vi "subAcquisition_zStack.vi"(6 "Ti-E cluster":T2, 7 "Z-stack cluster":T1={"Timelapse Acquired"=1, "File path"=path "C:/Users/ZouOptics/Desktop/TEST", "Z-Stack"={"Z end"=0.0, "Step Num"=1, "Step Size"=2.0, "Z0"=3471.0, "z-stack?"=FALSE}, "Frames to avg."=20, "Image Info Ref"=refnum, "Camera Ctrl"={"Chosen Camera"=0, "ROI selection"=0, "Live"=FALSE, "ROI define"=FALSE, "Snap"=FALSE, "ROI update"=FALSE, "ROI previous "=FALSE, "ROI"={"Bin"=2, "ROI"={"x offset"=256, "y offset"=256, "x width"=512, "y width"=512}}, "Exposure (ms)"=100.0, "Symmetrical"=FALSE, "Autoscale"=TRUE, "Scale"={"Scale.Min"=0, "Scale.Max"=6038}}} {"Camera Ctrl"."Scale"."Scale.Max" min=1 max=5000 step=1; "Camera Ctrl"."Scale"."Scale.Min" min=1 max=5000 step=1; "Camera Ctrl"."Exposure (ms)" min=1.0 max=5000.0 step=1.0; "Camera Ctrl"."ROI"."ROI"."x offset" min=1 max=512 step=1; "Camera Ctrl"."ROI"."ROI"."y offset" min=1 max=512 step=1; "Camera Ctrl"."ROI"."ROI"."x width" min=1 max=512 step=1; "Camera Ctrl"."ROI"."ROI"."y width" min=1 max=512 step=1; "Camera Ctrl"."ROI"."Bin" items=["1x1"=1, "2x2"=2, "4x4"=4]; "Camera Ctrl"."ROI selection" items=["Full ROI", "Central quad", "Confocal"]; "Camera Ctrl"."Chosen Camera" items=["Left", "Right"]}, 8 "error in":errorcluster, 10 "Z Stack Aquired Refnum":refnum<vi>, 11 "Handle in":u32) -> (0 "error out":errorcluster)   [LabVIEW 2015]
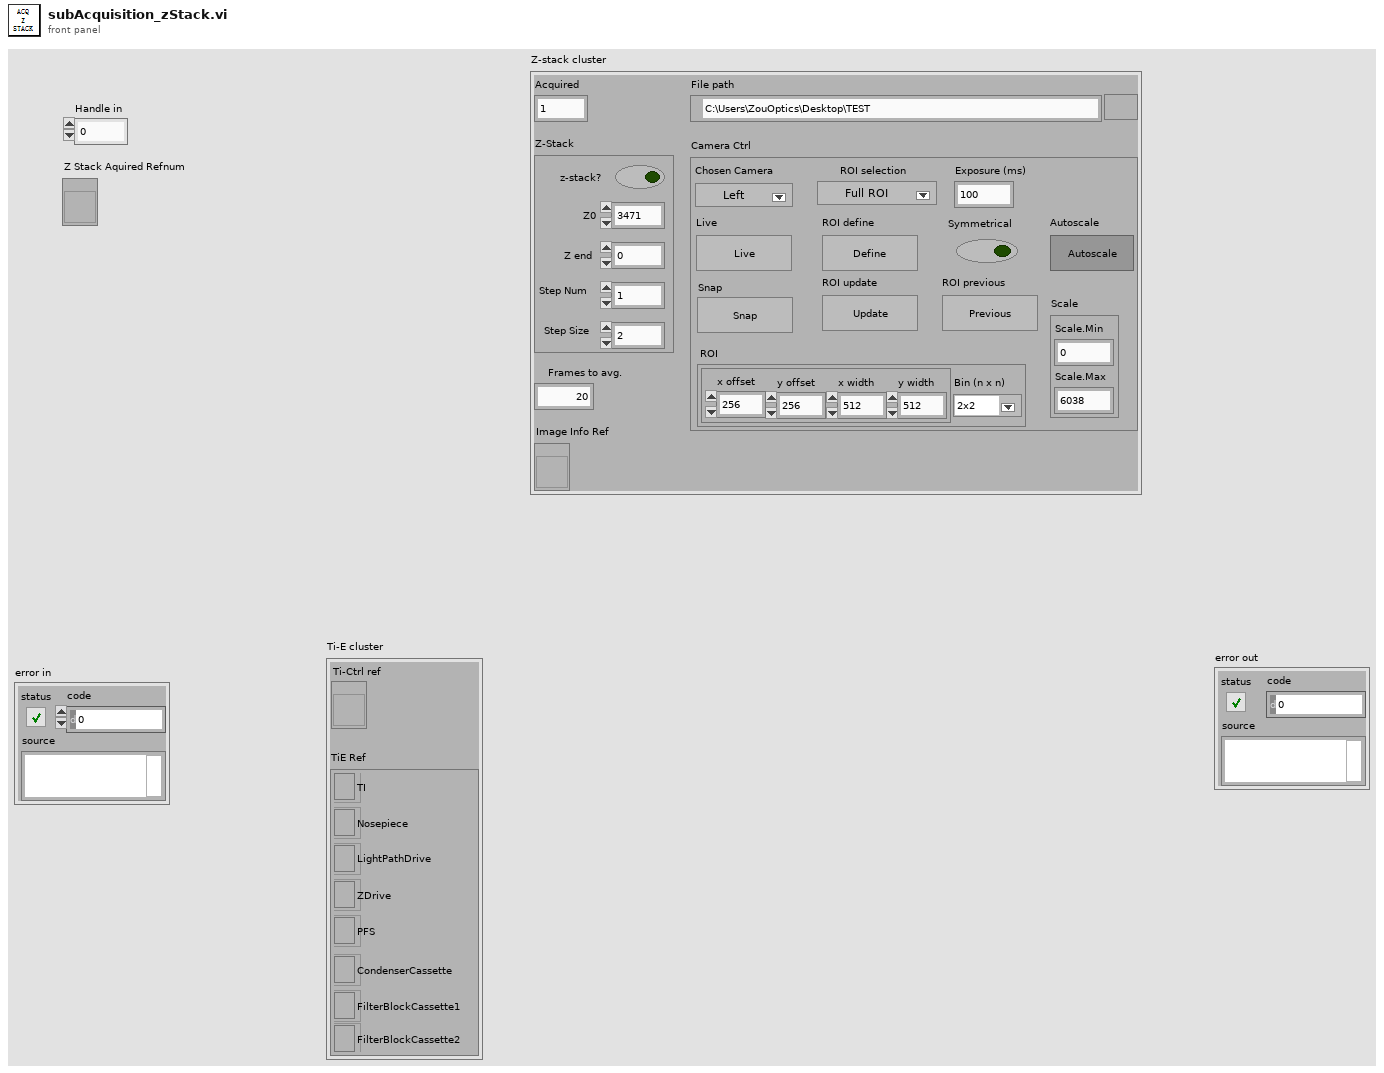
[diagram p1: front panel]
types:
  T1 = cluster{"Timelapse Acquired":i32, "File path":path, "Z-Stack":cluster{"Z end":dbl, "Step Num":i32, "Step Size":dbl, "Z0":dbl, "z-stack?":bool}, "Frames to avg.":i32, "Image Info Ref":refnum<vi>, "Camera Ctrl":cluster{"Chosen Camera":u32, "ROI selection":u16, "Live":bool, "ROI define":bool, "Snap":bool, "ROI update":bool, "ROI previous ":bool, "ROI":cluster{"Bin":u16, "ROI":cluster{"x offset":i32, "y offset":i32, "x width":i32, "y width":i32}}, "Exposure (ms)":dbl, "Symmetrical":bool, "Autoscale":bool, "Scale":cluster{"Scale.Min":i32, "Scale.Max":i32}}}
  T2 = cluster{"Ti-Ctrl ref":refnum<vi>, "TiE Ref":cluster{"TI":refnum<k7>, "Nosepiece":refnum<k7>, "LightPathDrive":refnum<k7>, "ZDrive":refnum<k7>, "PFS":refnum<k7>, "CondenserCassette":refnum<k7>, "FilterBlockCassette1":refnum<k7>, "FilterBlockCassette2":refnum<k7>}}
  T3 = cluster{"TI":refnum<k7>, "Nosepiece":refnum<k7>, "LightPathDrive":refnum<k7>, "ZDrive":refnum<k7>, "PFS":refnum<k7>, "CondenserCassette":refnum<k7>, "FilterBlockCassette1":refnum<k7>, "FilterBlockCassette2":refnum<k7>}
  T4 = enum8{"Enabled", "Disabled", "Disabled and Grayed Out"}
  T5 = cluster{"Bin":u16, "ROI":cluster{"x offset":i32, "y offset":i32, "x width":i32, "y width":i32}}
  T6 = cluster{"Status":string, "scale bar (μm)":dbl, "Image":u16[][], "Histogram":cluster{"max value":u16, "mean":i16, "min value":u16, "Histogram":cluster{"X Values":dbl[], "Histogram: h(x)":i32[]}}, "Scale Info":cluster{"Pixel size (nm)":dbl, "Total x width (μm)":dbl, "Total y width (μm)":dbl}, "Camera View indicator":u16[][], "max frame rate (Hz)":dbl}
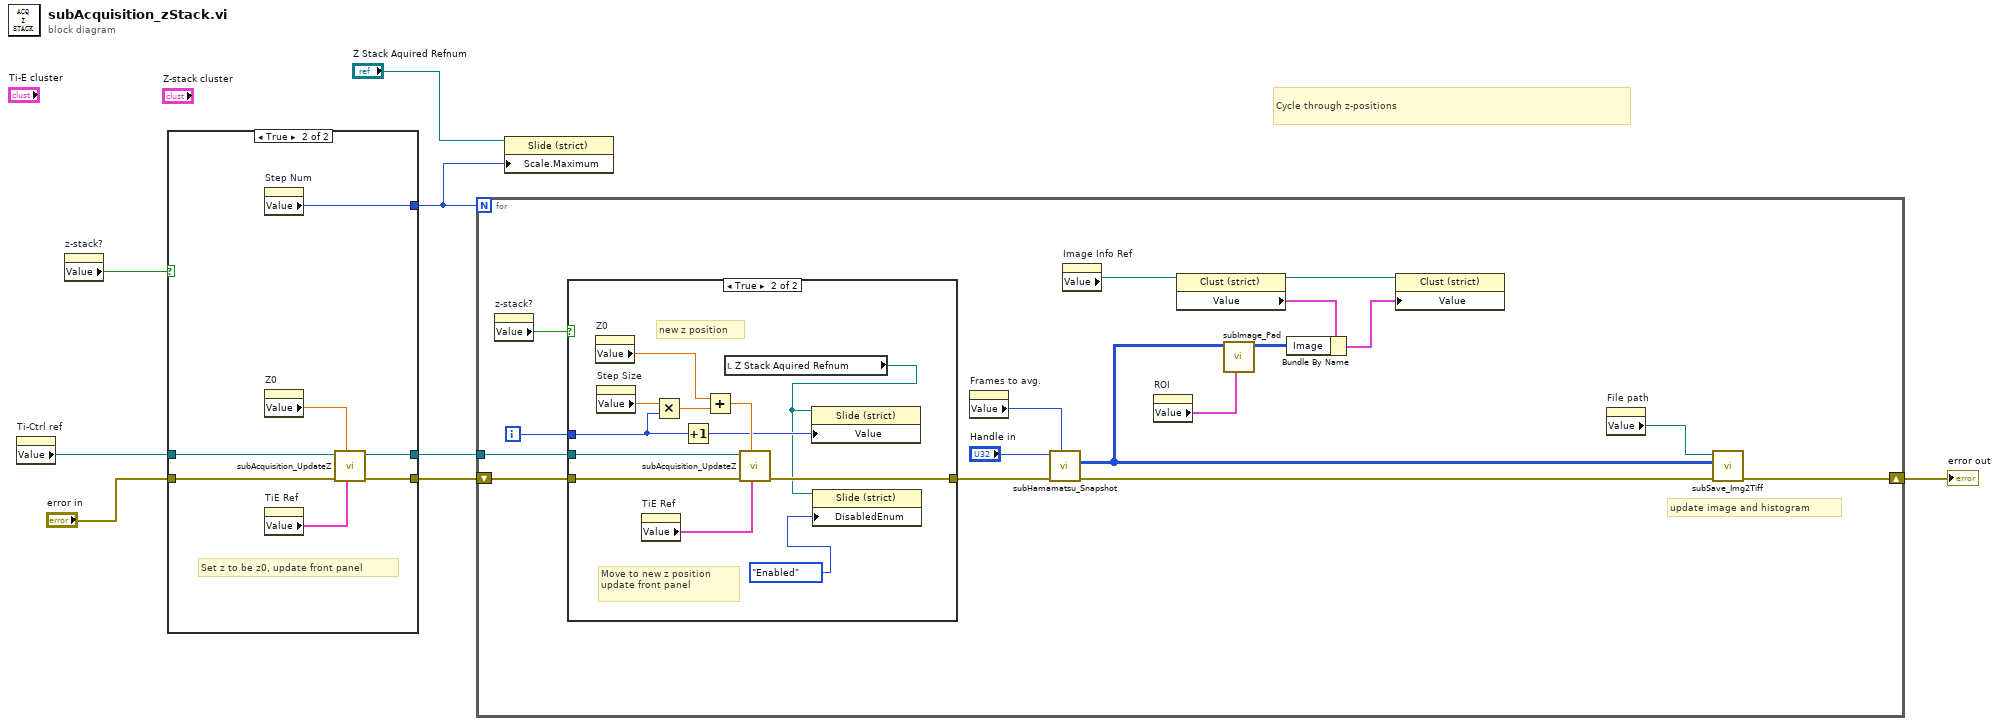
[diagram p0: block diagram]
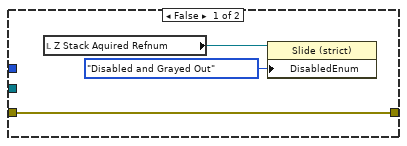
[diagram p2: hidden frame]
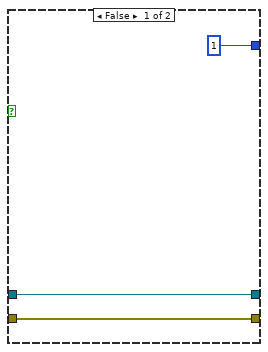
[diagram p3: hidden frame]
diagram:
  # "Cycle through z-positions"
  n1 = property on="Ti-Ctrl ref" class="LVObjRef (strict)"() -> ("Value"=w5:refnum<vi>)  [unwired: 2 in, 2 out]
  n2 = property on="z-stack?" class="Bool (strict)"() -> ("Value"=w4:bool)  [unwired: 2 in, 2 out]
  n3 = case shown="True" w4 {
    tunnel: "error in" -> [w11 w17]
    tunnel: [w11 w15] -> w7
    tunnel: [1 ("Step Num") w12] -> w2
    tunnel: w5 -> [w9 w18]
    tunnel: [w9 w16] -> w6
    frame False {
    }
    frame True {
      # "Set z to be z0, update front panel"
      n4 = property on="Step Num" class="DigNum (strict)"() -> ("Value"=w12:i32)  [unwired: 2 in, 2 out]
      n5 = property on="Z0" class="DigNum (strict)"() -> ("Value"=w13:dbl)  [unwired: 2 in, 2 out]
      n6 = property on="TiE Ref" class="Clust (strict)"() -> ("Value"=w14:T3)  [unwired: 2 in, 2 out]
      n7 = call "subAcquisition_UpdateZ.vi"("Ref"=w14, "z"=w13, "error in"=w17, "TiCtrl ref in"=w18) -> ("error out"=w15:errorcluster, "TiCtrl ref out"=w16:refnum<vi>)  [unwired: 6 in]
    }
  }
  n8 = for {
    N: w2 -> [_]
    shift-right: [w33] -> w3
    shift-left: w7 -> [w35]
    tunnel: w6 -> [w34]
    i -> [w30]
    # "update image and histogram"
    n9 = property on="z-stack?" class="Bool (strict)"() -> ("Value"=w19:bool)  [unwired: 2 in, 2 out]
    n10 = case shown="True" w19 {
      tunnel: w35 -> [w38 w50]
      tunnel: w34 -> [_ w48]
      tunnel: [w38 w47] -> w32
      tunnel: w30 -> [_ w42]
      frame False {
        n11 = local read "Z Stack Aquired Refnum"() -> (w37:refnum<vi>)
        n12 = property class="Slide (strict)"(reference=w37, "DisabledEnum"=T4."Disabled and Grayed Out" ("Disabled")) -> ()  [unwired: 1 in, 2 out]
      }
      frame True {
        # "Move to new z position\nupdate front panel"
        # "new z position"
        n13 = property on="Z0" class="DigNum (strict)"() -> ("Value"=w43:dbl)  [unwired: 2 in, 2 out]
        n14 = property on="Step Size" class="DigNum (strict)"() -> ("Value"=w44:dbl)  [unwired: 2 in, 2 out]
        n15 = property on="TiE Ref" class="Clust (strict)"() -> ("Value"=w46:T3)  [unwired: 2 in, 2 out]
        n16 = Multiply(x=w44, y=w42) -> (x*y=w45:dbl)
        n17 = Increment(x=w42) -> (x+1=w41:i32)
        n18 = Add(x=w43, y=w45) -> (x+y=w49:dbl)
        n19 = local read "Z Stack Aquired Refnum"() -> (w40:refnum<vi>)
        n20 = call "subAcquisition_UpdateZ.vi"("Ref"=w46, "z"=w49, "error in"=w50, "TiCtrl ref in"=w48) -> ("error out"=w47:errorcluster)  [unwired: 6 in, 1 out]
        n21 = property class="Slide (strict)"(reference=w40, "Value"=w41) -> ()  [unwired: 1 in, 2 out]
        n22 = property class="Slide (strict)"(reference=w40, "DisabledEnum"=T4."Enabled" ("Disabled")) -> ()  [unwired: 1 in, 2 out]
      }
    }
    n23 = property on="Frames to avg." class="DigNum (strict)"() -> ("Value"=w29:i32)  [unwired: 2 in, 2 out]
    n24 = call "subHamamatsu_Snapshot.vi"("Frames to average (1)"=w29, "Error in"=w32, "Value"="Handle in") -> ("Error out"=w31:errorcluster, "Image"=w24:u16[][])  [unwired: 6 in, 1 out]
    n25 = property on="Image Info Ref" class="LVObjRef (strict)"() -> ("Value"=w25:refnum<vi>)  [unwired: 2 in, 2 out]
    n26 = property on="ROI" class="Clust (strict)"() -> ("Value"=w20:T5)  [unwired: 2 in, 2 out]
    n27 = property class="Clust (strict)"(reference=w25) -> (reference out=w28:refnum<vi>, "Value"=w22:T6)  [unwired: 1 in, 1 out]
    n28 = call "subImage_Pad.vi"("ROI"=w20, "Image in"=w24) -> ("Image out"=w23:u16[][])  [unwired: 7 in, 2 out]
    n29 = Bundle By Name(cluster=w22, "Image"=w23) -> (w21:T6)
    n30 = property class="Clust (strict)"(reference=w28, "Value"=w21) -> ()  [unwired: 1 in, 2 out]
    n31 = property on="File path" class="Path"() -> ("Value"=w26:path)  [unwired: 2 in, 2 out]
    n32 = call "subSave_Img2Tiff.vi"("Error in (no error)"=w31, "Image"=w24, "File path/name"=w26) -> ("Error out"=w33:errorcluster)  [unwired: 7 in, 1 out]
  }
  "error out" <- w3
  n33 = property class="Slide (strict)"(reference="Z Stack Aquired Refnum", "Scale.Maximum"=w2) -> ()  [unwired: 1 in, 2 out]
